vi "Initialize.vi"(7 "Serial Settings":T1={"Baud Rate (9600)"=9600, "Flow Control (RTS/CTS)"=2, "Data Bits (8)"=8} {"Flow Control (RTS/CTS)" items=["None"=0, "RTS/CTS"=2]; "Baud Rate (9600)" items=["1200"=1200, "2400"=2400, "4800"=4800, "9600"=9600, "19200"=19200, "38400"=38400]}, 8 "error in (no error)":errorcluster {"code" format="%.0x"}, 9 "ID Query (T: Query)":bool=TRUE, 10 "Reset Device (T: Reset)":bool=TRUE, 11 "VISA Resource Name":refnum<visa-resource-name>="GPIB0::1::INSTR") -> (0 "error out":errorcluster {"code" format="%.0x"}, 3 "VISA Resource Name Out":refnum<visa-resource-name>)   [LabVIEW 2010, in "Tektronix TDS 3000 Series.lvlib"]
doc: "Passes the addressing information in the instrument resource name to the VISA Open VI and returns the instrument ID.\n\nNote: \n (1) This instrument driver supports serial communication. If problems are encountered when using serial communication, recommend using baud rates less than 19,200, hardware handshaking, and increase the delay time of tktds3k VISA write and clear VIs. National Instruments does not provide technical support for the oscilloscope’s physical serial interface. National Instruments will support driver related issues. If you need technical support related to the physical serial interface on either the TDS 30xx series please contact Tektronix\n\n(2) If using the serial interface to communicate with your instrument, it is required that you use RTS CTS Flow control (Hardflagging Flow Control). If you do wish to use the serial interface, set the serial settings on the instrument to be the same as the serial settings on the block diagram:\n\nBaud rate = 9600 (Faster Baud Rate can be used upto 38400)\nParity = NONE (0)\nData bits = 8\nFlow control = Flow RTS CTS (Hard Flagging) (2)\nStop bits = Stop One (10)\nTermination character (EOL String) = LF (\"\\n\")\n\n(3) This instrument supports ethernet connections. Make sure the instrument is correctly set up to the network before trying to connect to it."
uses:
  <instrlib>/Tektronix TDS 3000 Series/Tektronix TDS 3000 Series.lvlib
panel:
  # "© 2003-2006, National Instruments, Corporation.  All Rights Reserved."
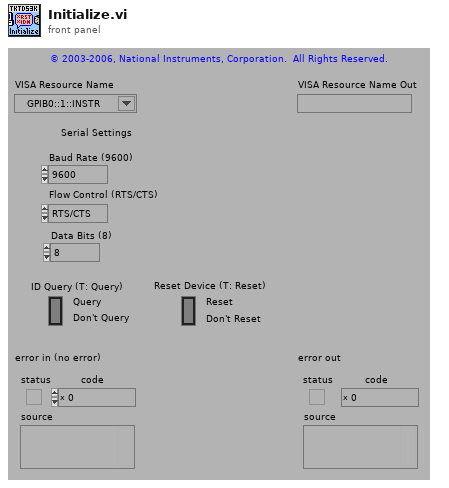
[diagram p1: front panel]
types:
  T1 = cluster{"Baud Rate (9600)":u32, "Flow Control (RTS/CTS)":u16, "Data Bits (8)":u16}
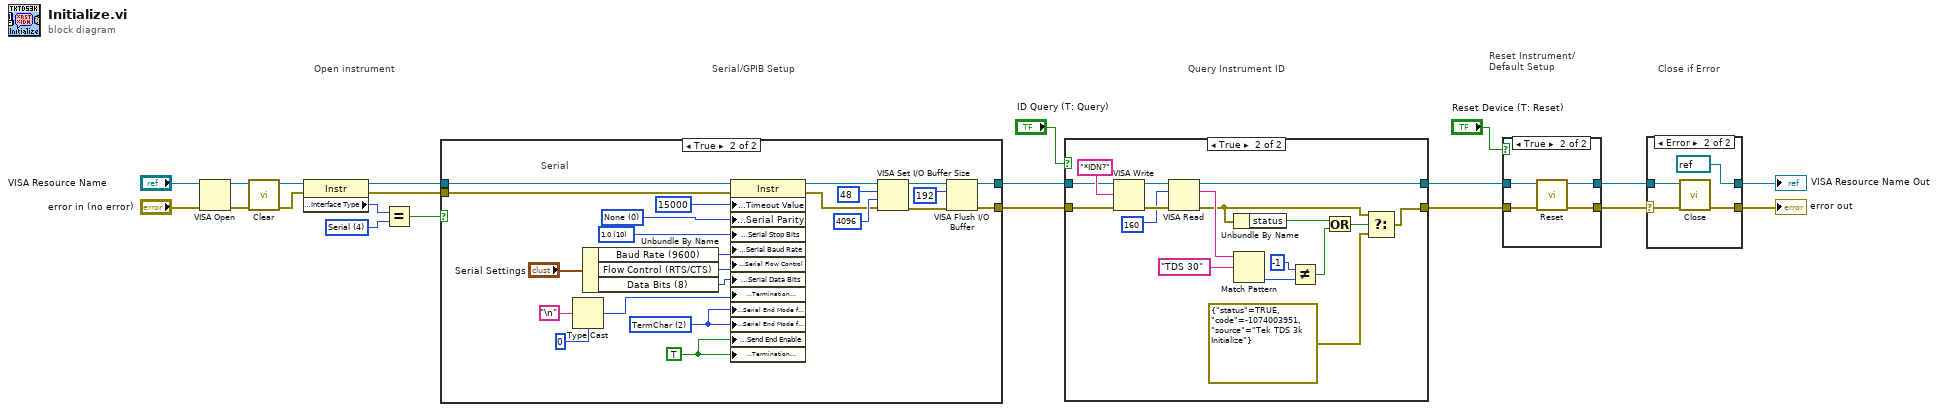
[diagram p0: block diagram]
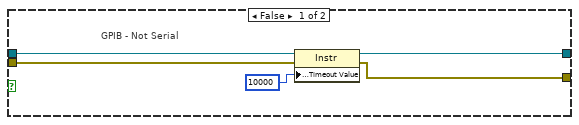
[diagram p3: hidden frame]
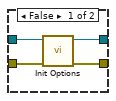
[diagram p5: hidden frame]
diagram:
  w3 = u16 4 items=["GPIB"=1, "VXI"=2, "GPIB-VXI"=3, "Serial"=4, "PXI"=5, "TCPIP"=6, "USB"=7] ("Interface Information:Interface Type")
  # "Serial/GPIB Setup"
  # "Close if Error"
  # "Reset Instrument/\nDefault Setup"
  # "Open instrument"
  # "Query Instrument ID"
  n1 = VISA Open(error in (no error)="error in (no error)", VISA resource name="VISA Resource Name") -> (VISA resource name=w10:refnum<visa-resource-name>, error out=w9:errorcluster)  [unwired: 3 in]
  n2 = call <instrlib>:"Clear.vi"("error in (no error)"=w9, "VISA Resource Name"=w10) -> ("error out"=w5:errorcluster, "VISA Resource Name Out"=w8:refnum<visa-resource-name>)  [unwired: 8 in]
  n3 = property class="Instr"(reference=w8, error in=w5) -> (reference out=w7:refnum<visa-resource-name>, error out=w6:errorcluster, "Interface Information:Interface Type"=w4:u16)
  n4 = Equal?(x=w4, y=w3) -> (x = y?=w2:bool)
  n5 = case shown="True" w2 {
    tunnel: w7 -> [w26 w34]
    tunnel: w6 -> [w25 w33]
    tunnel: [w24 w44] -> w14
    tunnel: [w23 w43] -> w13
    frame False {
      # "GPIB - Not Serial"
      n6 = property class="Instr"(reference=w26, error in=w25, "General Settings:Timeout Value"=u32 10000) -> (reference out=w24:refnum<visa-resource-name>, error out=w23:errorcluster)
    }
    frame True {
      w37 = u16 10 items=["1.0"=10, "1.5"=15, "2.0"=20] ("Serial Settings:Serial Stop Bits")
      w36 = u16 0 items=["None", "Odd", "Even", "Mark", "Space"] ("Serial Settings:Serial Parity")
      w29 = u16 2 items=["None", "LastBit", "TermChar"] ("Serial Settings:Serial End Mode for Reads")
      w30 = TRUE ("Message Based Settings:Termination Character Enable")
      # "Serial"
      n7 = Type Cast(type=u8 0, x="\n") -> (*(type *) &x=w28:u8)
      n8 = Unbundle By Name("Serial Settings") -> ("Baud Rate (9600)"=w39:u32, "Flow Control (RTS/CTS)"=w40:u16, "Data Bits (8)"=w27:u16)
      n9 = property class="Instr"(reference=w34, error in=w33, "General Settings:Timeout Value"=u32 15000, "Serial Settings:Serial Parity"=w36, "Serial Settings:Serial Stop Bits"=w37, "Serial Settings:Serial Baud Rate"=w39, "Serial Settings:Serial Flow Control"=w40, "Serial Settings:Serial Data Bits"=w27, "Message Based Settings:Termination Character"=w28, "Serial Settings:Serial End Mode for Reads"=w29, "Serial Settings:Serial End Mode for Writes"=w29, "Message Based Settings:Send End Enable"=w30, "Message Based Settings:Termination Character Enable"=w30) -> (reference out=w31:refnum<visa-resource-name>, error out=w32:errorcluster)
      n10 = VISA Set I/O Buffer Size(VISA resource name=w31, mask (16)=u16 48, size (4096)=u32 4096, error in (no error)=w32) -> (VISA resource name out=w46:refnum<visa-resource-name>, error out=w45:errorcluster)
      n11 = VISA Flush I/O Buffer(VISA resource name=w46, mask (16)=u16 192, error in (no error)=w45) -> (VISA resource name out=w44:refnum<visa-resource-name>, error out=w43:errorcluster)
    }
  }
  n12 = case shown="True" "ID Query (T: Query)" {
    tunnel: [w50 w56] -> w17
    tunnel: w13 -> [w50 w60]
    tunnel: [w51 w63] -> w18
    tunnel: w14 -> [w51 w66]
    frame False {
    }
    frame True {
      n13 = VISA Write(VISA resource name=w66, write buffer="*IDN?", error in (no error)=w60) -> (VISA resource name out=w61:refnum<visa-resource-name>, error out=w65:errorcluster)  [unwired: 1 out]
      n14 = VISA Read(VISA resource name=w61, byte count=u32 160, error in (no error)=w65) -> (VISA resource name out=w63:refnum<visa-resource-name>, read buffer=w64:string, error out=w58:errorcluster)  [unwired: 1 out]
      n15 = Unbundle By Name(w58) -> ("status"=w57:bool)
      n16 = Match Pattern(string=w64, regular expression="TDS 30") -> (offset past match=w54:i32)  [unwired: 1 in, 3 out]
      n17 = Not Equal?(x=-1, y=w54) -> (x != y?=w53:bool)
      n18 = Or(x=w57, y=w53) -> (x .or. y?=w59:bool)
      n19 = Select(t=w58, s=w59, f=errorcluster {"status"=TRUE, "code"=-1074003951, "source"="Tek TDS 3k Initialize"} ("error out")) -> (s? t:f=w56:errorcluster)
    }
  }
  n20 = case shown="True" "Reset Device (T: Reset)" {
    tunnel: w17 -> [w70 w75]
    tunnel: [w71 w73] -> w1
    tunnel: w18 -> [w69 w76]
    tunnel: [w72 w74] -> w19
    frame False {
      n21 = call <instrlib>:"Init Options.vi"("error in (no error)"=w70, "VISA Resource Name"=w69) -> ("error out"=w71:errorcluster, "VISA Resource Name Out"=w72:refnum<visa-resource-name>)  [unwired: 8 in]
    }
    frame True {
      n22 = call <instrlib>:"Reset.vi"("error in (no error)"=w75, "VISA Resource Name"=w76) -> ("error out"=w73:errorcluster, "VISA Resource Name Out"=w74:refnum<visa-resource-name>)  [unwired: 8 in]
    }
  }
  n23 = case shown="Error" w1 {
    selector: w1 -> [w77 w80]
    tunnel: w19 -> [w78 w81]
    tunnel: [w78 refnum<visa-resource-name> refnum ("dup VISA session")] -> w12
    tunnel: [w77 w82] -> w11
    frame No Error {
    }
    frame Error {
      n24 = call <instrlib>:"Close.vi"("error in (no error)"=w80, "VISA Resource Name"=w81) -> ("error out"=w82:errorcluster)  [unwired: 9 in]
    }
  }
  "error out" <- w11
  "VISA Resource Name Out" <- w12
